vi "OP300ZP_Test_DataDyn.vi"(4 "Vcell Max (V)":dbl, 5 "MCU":bool, 6 "Vcell Min (V)":dbl, 8 "errin":errorcluster, 9 "Température usine (°C)":dbl, 10 "Tcell Max (°C)":dbl, 11 "Tcell Min (°C)":dbl) -> (0 "errout":errorcluster, 1 "StrData":T1, 2 "datalog":string, 3 "pass":bool)   [LabVIEW 2020]
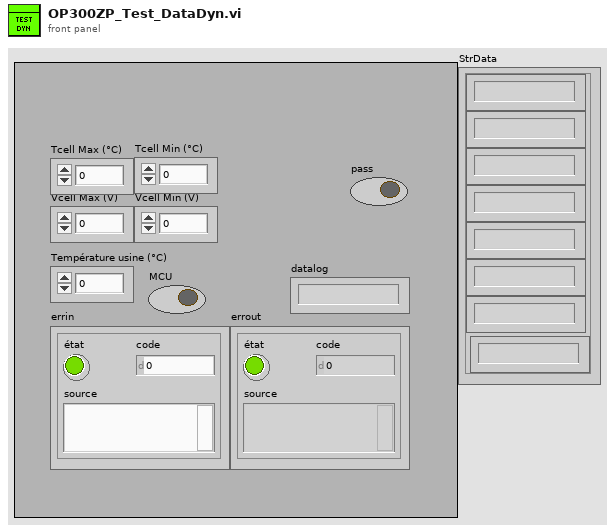
[diagram p1: front panel]
types:
  T1 = cluster{"Chaîne":string, "Chaîne":string, "Chaîne":string, "Chaîne":string, "Chaîne":string, "Chaîne":string, "Chaîne":string, "Chaîne 2":string}
  T2 = cluster{string, string, string, string, string, string, string, "cas vrai":string}
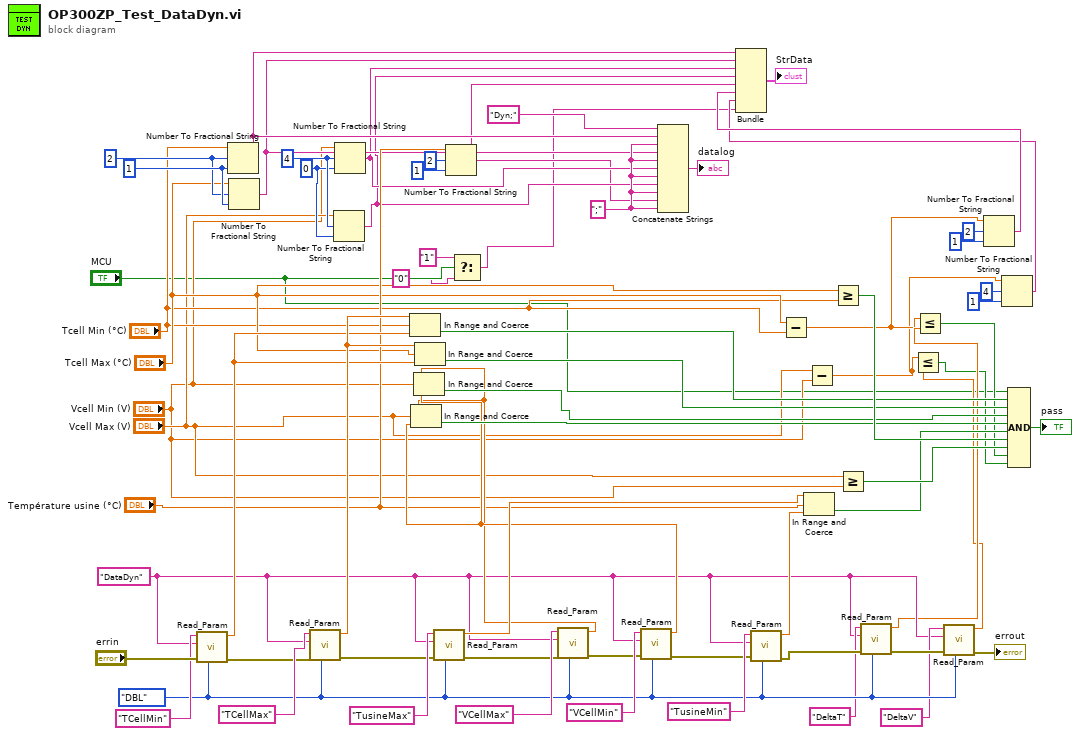
[diagram p0: block diagram]
diagram:
  w35 = ";" ("chaîne")
  w39 = i16 0 ("précision (6)")
  w40 = i16 4 ("largeur (-)")
  w42 = i16 1 ("précision (6)")
  w41 = i16 2 ("largeur (-)")
  w25 = enum16{"STR", "DBL", "U32"}."DBL" ("Énum")
  w22 = "DataDyn" ("section")
  n1 = call "Read_Param.vi"("Énum"=w25, "errin"="errin", "section"=w22, "key"="TCellMin") -> ("error out"=w44:errorcluster, "dbl"=w50:dbl)  [unwired: 3 in, 3 out]
  n2 = Number To Fractional String(number="Tcell Min (°C)", width (-)=w41, precision (6)=w42) -> (F-format string=w33:string)  [unwired: 1 in]
  n3 = Number To Fractional String(number="Tcell Max (°C)", width (-)=w41, precision (6)=w42) -> (F-format string=w32:string)  [unwired: 1 in]
  n4 = call "Read_Param.vi"("Énum"=w25, "errin"=w44, "section"=w22, "key"="TCellMax") -> ("error out"=w45:errorcluster, "dbl"=w52:dbl)  [unwired: 3 in, 3 out]
  n5 = Number To Fractional String(number="Vcell Max (V)", width (-)=w40, precision (6)=w39) -> (F-format string=w30:string)  [unwired: 1 in]
  n6 = Number To Fractional String(number="Vcell Min (V)", width (-)=w40, precision (6)=w39) -> (F-format string=w31:string)  [unwired: 1 in]
  n7 = In Range and Coerce(upper limit=w52, x="Tcell Min (°C)", lower limit=w50) -> (In Range?=w61:bool)  [unwired: 1 out]
  n8 = In Range and Coerce(upper limit=w52, x="Tcell Max (°C)", lower limit=w50) -> (In Range?=w62:bool)  [unwired: 1 out]
  n9 = call "Read_Param.vi"("Énum"=w25, "errin"=w45, "section"=w22, "key"="TusineMax") -> ("error out"=w46:errorcluster, "dbl"=w57:dbl)  [unwired: 3 in, 3 out]
  n10 = Number To Fractional String(number="Température usine (°C)", width (-)=i16 2 ("largeur (-)"), precision (6)=i16 1 ("précision (6)")) -> (F-format string=w29:string)  [unwired: 1 in]
  n11 = Select(t="1" ("cas vrai"), s="MCU", f="0") -> (s? t:f=w1:string)
  n12 = call "Read_Param.vi"("Énum"=w25, "errin"=w46, "section"=w22, "key"="VCellMax") -> ("error out"=w47:errorcluster, "dbl"=w54:dbl)  [unwired: 3 in, 3 out]
  n13 = call "Read_Param.vi"("Énum"=w25, "errin"=w47, "section"=w22, "key"="VCellMin") -> ("error out"=w48:errorcluster, "dbl"=w55:dbl)  [unwired: 3 in, 3 out]
  n14 = In Range and Coerce(upper limit=w54, x="Vcell Max (V)", lower limit=w55) -> (In Range?=w64:bool)  [unwired: 1 out]
  n15 = In Range and Coerce(upper limit=w54, x="Vcell Min (V)", lower limit=w55) -> (In Range?=w63:bool)  [unwired: 1 out]
  n16 = Concatenate Strings("Dyn;" ("chaîne"), w33, w35, w32, w35, w31, w35, w30, w35, w29, w35) -> (→"datalog":string)
  n17 = call "Read_Param.vi"("Énum"=w25, "errin"=w48, "section"=w22, "key"="TusineMin") -> ("error out"=w28:errorcluster, "dbl"=w58:dbl)  [unwired: 3 in, 3 out]
  n18 = Subtract(x="Tcell Max (°C)", y="Tcell Min (°C)") -> (x-y=w9:dbl)
  n19 = In Range and Coerce(upper limit=w57, x="Température usine (°C)", lower limit=w58) -> (In Range?=w65:bool)  [unwired: 1 out]
  n20 = Subtract(x="Vcell Max (V)", y="Vcell Min (V)") -> (x-y=w6:dbl)
  n21 = Greater Or Equal?(x="Tcell Max (°C)", y="Tcell Min (°C)") -> (x >= y?=w66:bool)
  n22 = Greater Or Equal?(x="Vcell Max (V)", y="Vcell Min (V)") -> (x >= y?=w67:bool)
  n23 = call "Read_Param.vi"("Énum"=w25, "errin"=w28, "section"=w22, "key"="DeltaT") -> ("error out"=w27:errorcluster, "dbl"=w17:dbl)  [unwired: 3 in, 3 out]
  n24 = Less Or Equal?(x=w9, y=w17) -> (x <= y?=w15:bool)
  n25 = call "Read_Param.vi"("Énum"=w25, "errin"=w27, "section"=w22, "key"="DeltaV") -> ("error out"=→"errout":errorcluster, "dbl"=w16:dbl)  [unwired: 3 in, 3 out]
  n26 = Less Or Equal?(x=w6, y=w16) -> (x <= y?=w14:bool)
  n27 = Number To Fractional String(number=w9, width (-)=i16 2 ("largeur (-)"), precision (6)=i16 1 ("précision (6)")) -> (F-format string=w8:string)  [unwired: 1 in]
  n28 = Number To Fractional String(number=w6, width (-)=i16 4 ("largeur (-)"), precision (6)=i16 1 ("précision (6)")) -> (F-format string=w7:string)  [unwired: 1 in]
  n29 = Bundle(w33, w32, w31, w30, w29, w8, w7, "cas vrai"=w1) -> (→"StrData":T2)  [unwired: 1 in]
  n30 = Compound Arithmetic op=AND ("Opérateur arithmétique")("MCU", w61, w62, w63, w64, w65, w66, w67, w15, w14) -> (→"pass":bool)
